vi "Actor Core.vi"(8 "error in":errorcluster, 11 "Master Controller in":refnum<class "Master Controller.lvclass">) -> (0 "error out":errorcluster, 3 "Actor out":refnum<class "Actor.lvclass">)   [LabVIEW 2015, in "Master Controller Core.lvlib" / "Master Controller.lvclass"]
doc: "(<B>Filename</B>: Actor Framework.lvlib:Actor.lvclass:Actor Core.vi)\n\nReceives messages to the actor, reacts to them, and initiates any error handling that may shut the actor down.\n\nDescendant classes may override this VI to append parallel tasks for the actor to complete while it handles messages. Overrides use the Call Parent Method node."
uses:
  Master Controller.lvclass
  <vilib>/ActorFramework/Actor/Actor.lvclass
  Utilities/Status Messaging.llb/Status Message Command.ctl
  <vilib>/ActorFramework/Actor/Actor.lvclass/Actor.ctl
  <vilib>/ActorFramework/Message Enqueuer/Message Enqueuer.lvclass/Message Enqueuer.ctl
  <vilib>/ActorFramework/Message Enqueuer/Init from Existing Queue.vi
  <vilib>/ActorFramework/Message Enqueuer/Enqueue.vi
  <vilib>/ActorFramework/Message Priority Queue/Priority Enqueue.vi
  <vilib>/ActorFramework/Message Enqueuer/Message Enqueuer.lvclass
  <vilib>/ActorFramework/Stop Msg/Stop Msg.lvclass
  Utilities/Status Messaging.llb/Status Messaging.lvlib
panel:
  out "Status":string
  in  "stop":bool
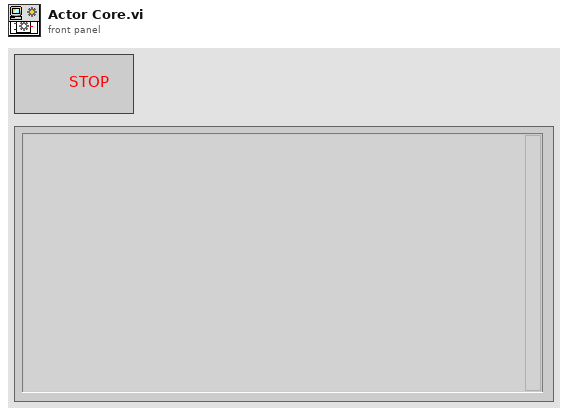
[diagram p1: front panel]
types:
  T1 = typedef "Status Messaging.lvlib/Status Message Command.ctl" = enum16{"Write", "Obtain", "Kill"}
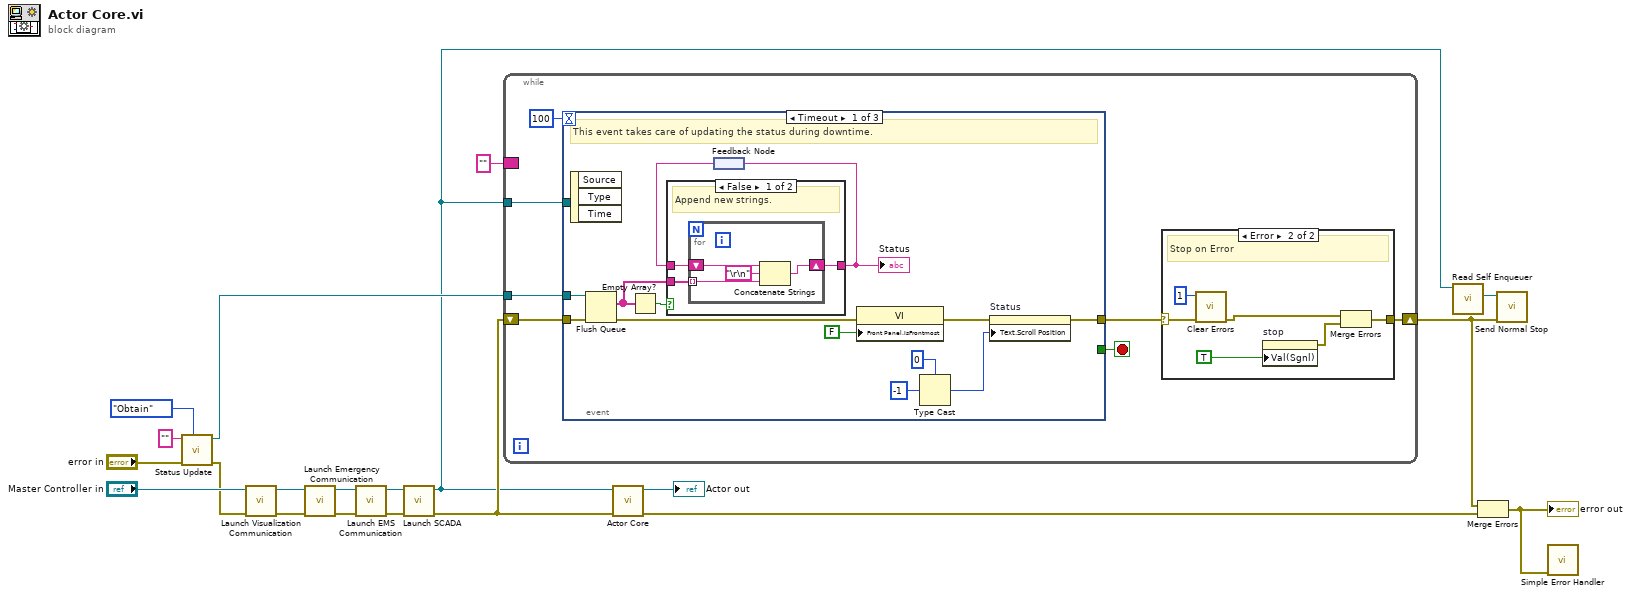
[diagram p0: block diagram]
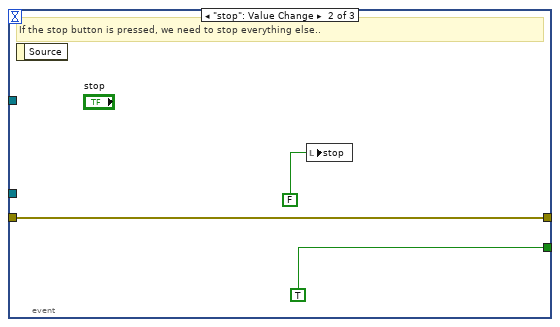
[diagram p4: hidden frame]
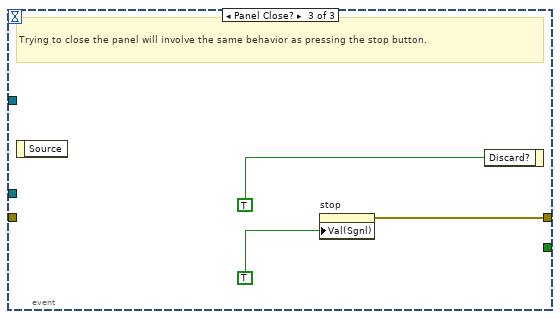
[diagram p5: hidden frame]
diagram:
  n1 = call "Status Update.vi"("Command (Write)"=Status_Message_Command."Obtain", "error in (no error)"="error in", "Status Update"="") -> ("error out"=w9:errorcluster, "queue out"=w7:refnum<queue>)  [unwired: 7 in]
  n2 = call "Launch Visualization Communication.vi"("error in (no error)"=w9, "Master Controller in"="Master Controller in") -> ("error out"=w13:errorcluster, "Master Controller out"=w14:refnum<class "Master Controller.lvclass">)  [unwired: 8 in]
  n3 = call "Launch Emergency Communication.vi"("error in (no error)"=w13, "Master Controller in"=w14) -> ("error out"=w17:errorcluster, "Master Controller out"=w16:refnum<class "Master Controller.lvclass">)  [unwired: 8 in]
  n4 = call "Launch EMS Communication.vi"("error in (no error)"=w17, "Master Controller in"=w16) -> ("error out"=w18:errorcluster, "Master Controller out"=w19:refnum<class "Master Controller.lvclass">)  [unwired: 8 in]
  n5 = call "Launch SCADA.vi"("error in (no error)"=w18, "Master Controller in"=w19) -> ("error out"=w6:errorcluster, "Master Controller out"=w1:refnum<class "Master Controller.lvclass">)  [unwired: 8 in]
  n6 = while {
    tunnel: w7 -> [w26]
    border: "" ("Status") -> [_]
    shift-right: [w21] -> w2
    shift-left: w6 -> [w25]
    tunnel: w1 -> [w24]
    stop <- w23 stop-if-true
    n7 = event shown="[0] Timeout" {
      selector: _ -> [_ _ _]
      dyn-events: _ -> [_ _ _]
      timeout: 100 -> [_ _ _]
      tunnel: w26 -> [w47 _ _]
      tunnel: w25 -> [w44 w57 _]
      tunnel: w24 -> [_ _ _]
      tunnel: [_ TRUE _] -> w23
      tunnel: [w35 w57 w61] -> w22
      event Timeout {
        # "This event takes care of updating the status during downtime."
        n8 = event-data() -> ()  [unwired: 1 in, 3 out]
        n9 = Flush Queue(queue=w47, error in (no error)=w44) -> (remaining elements=w42:string[], error out=w40:errorcluster)  [unwired: 1 out]
        n10 = Empty Array?(array=w42) -> (empty?=w43:bool)
        n11 = feedback #1() -> (w46:string)
        n12 = case shown="False" w43 {
          tunnel: w46 -> [w49 w55]
          tunnel: [w48 w55] -> w45
          tunnel: w42 -> [w50 _]
          frame False {
            # "Append new strings."
            n13 = for {
              tunnel: w50 -> [w52] mode=indexing
              shift-right: [w51] -> w48
              shift-left: w49 -> [w53]
              n14 = Concatenate Strings(w53, "\r\n", w52) -> (w51:string)
            }
          }
          frame True, Default {
            # "Don't add empty strings."
          }
        }
        "Status" <- w45
        n15 = feedback-in #1(w45) -> ()
        n16 = property class="VI"(error in=w40, "Front Panel.IsFrontmost"=FALSE ("Front Panel Window:Is Frontmost")) -> (error out=w36:errorcluster)  [unwired: 1 in, 1 out]
        n17 = Type Cast(type=u32 0 ("Text.Scroll Position"), x=-1) -> (*(type *) &x=w37:u32)
        n18 = property on="Status" class="Str"(error in=w36, "Text.Scroll Position"=w37) -> (error out=w35:errorcluster)  [unwired: 1 in, 1 out]
      }
      event "stop": Value Change {
        # "If the stop button is pressed, we need to stop everything else.."
        n19 = event-data() -> ()  [unwired: 1 in, 1 out]
        n20 = local write "stop"(FALSE ("stop")) -> ()
      }
      event Panel Close? {
        # "Trying to close the panel will involve the same behavior as pressing the stop button."
        n21 = event-data() -> ()  [unwired: 1 in, 1 out]
        n22 = property on="stop" class="Bool (strict)"("Val(Sgnl)"=TRUE ("Discard?")) -> (error out=w61:errorcluster)  [unwired: 2 in, 1 out]
        n23 = event-data("Discard?"=TRUE) -> ()  [unwired: 1 in, 1 out]
      }
    }
    n24 = case shown="Error" w22 {
      selector: w22 -> [w28 w33]
      tunnel: [w28 w31] -> w21
      frame No Error {
      }
      frame Error {
        # "Stop on Error"
        n25 = call <vilib>:"Clear Errors.vi"("error in (no error)"=w33, "specific error code to clear (0: all)"=1) -> ("error out"=w30:errorcluster)  [unwired: 4 in, 1 out]
        n26 = property on="stop" class="Bool (strict)"("Val(Sgnl)"=TRUE ("Discard?")) -> (error out=w34:errorcluster)  [unwired: 2 in, 1 out]
        n27 = Merge Errors(w30, w34) -> (w31:errorcluster)
      }
    }
  }
  n28 = call-parent "Actor Core.vi"("error in"=w6, "Actor in"=w1) -> ("error out"=w15:errorcluster, "Actor out"=→"Actor out":refnum<class "Actor.lvclass">)  [unwired: 8 in]
  n29 = call <vilib>:"Read Self Enqueuer.vi"("Actor"=w1) -> ("Self Enqueuer"=w3:refnum<class "Message Enqueuer.lvclass">)  [unwired: 10 in]
  n30 = Merge Errors(w2, w15) -> (w4:errorcluster)
  "error out" <- w4
  n31 = call <vilib>:"Send Normal Stop.vi"("error in (no error)"=w2, "Message Enqueuer"=w3) -> ()  [unwired: 9 in, 1 out]
  n32 = call <vilib>:"Simple Error Handler.vi"("error in (no error)"=w4) -> ()  [unwired: 4 in, 5 out]
